vi "climb with joysticks.vi"   [LabVIEW 2012]
uses:
  <vilib>/Rock Robotics/WPI/Solenoid/WPI_SolenoidValue.ctl
  Robot Global Data.vi
  <vilib>/Rock Robotics/WPI/Solenoid/WPI_SolenoidSetEnum.vi
types:
  T1 = typedef "WPI_JoystickButtonState.ctl" = cluster{"Button 1":bool, "Button 2":bool, "Button 3":bool, "Button 4":bool, "Button 5":bool, "Button 6":bool, "Button 7":bool, "Button 8":bool, "Button 9":bool, "Button 10":bool, "Button 11":bool, "Button 12":bool}
  T2 = typedef "WPI_SolenoidValue.ctl" = enum16{"Off", "On", "Forward", "Reverse"}
  T3 = typedef "WPI_SolenoidDevRef.ctl" = cluster{"DevStatus":errorcluster, "Solenoid Module":T4, "Forward Solenoid Channel":T5, "Reverse Solenoid Channel":T5}
  T4 = typedef "FPGA_TypedefSolenoidModule.ctl" = enum16{"Solenoid Module 1", "Solenoid Module 2"}
  T5 = typedef "WPI_SolenoidChannel.ctl" = enum8{"Solenoid 1", "Solenoid 2", "Solenoid 3", "Solenoid 4", "Solenoid 5", "Solenoid 6", "Solenoid 7", "Solenoid 8", "Invalid"}
  T6 = typedef "WPI_MotorControlDeviceRef.ctl" = cluster{"DeviceStatus":errorcluster, "Type":enum16{"PWM", "CAN"}, "PWM":cluster{"Digital Module":T7, "PWM Channel":T8, "DeadBand":T9}, "CAN":cluster{"Device Number":u8, "Control Mode":T10, "Semaphore":T11, "Max Vout":dbl}, "Invert":bool, "TransformRef":T12, "InvTransformRef":T12}
  T7 = typedef "FPGA_TypedefDigitalModule.ctl" = enum16{"Digital Module 1", "Digital Module 2"}
  T8 = typedef "FPGA_DIOPWMChannel.ctl" = enum8{"PWM 1", "PWM 2", "PWM 3", "PWM 4", "PWM 5", "PWM 6", "PWM 7", "PWM 8", "PWM 9", "PWM 10", "Invalid"}
  T9 = typedef "WPI_PWMDeadband.ctl" = cluster{"Name":string, "maxPositivePwm":i32, "minPositivePwm":i32, "centerPwm":i32, "maxNegativePwm":i32, "minNegativePwm":i32, "angularRange":u16}
  T10 = typedef "WPI_CANJaguar_ControlMode.ctl" = enum8{"Percent VBus", "Current", "Speed", "Position", "Voltage"}
  T11 = typedef "Semaphore RefNum" = refnum<k1>
  T12 = typedef "WPI_PWMTransform_ConPane.ctl" = refnum<vi>
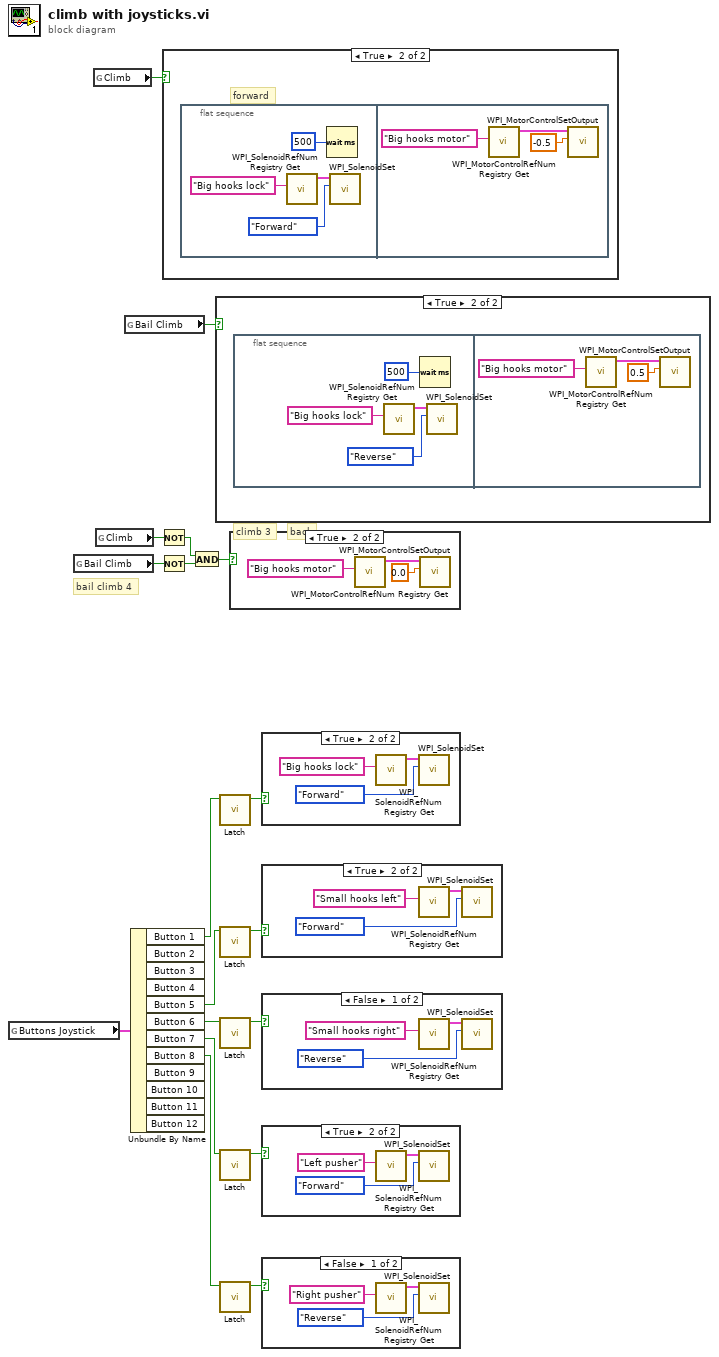
[diagram p0: block diagram]
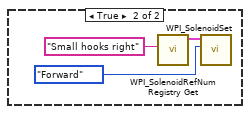
[diagram p2: hidden frame]
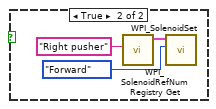
[diagram p3: hidden frame]
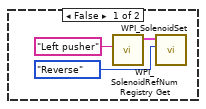
[diagram p4: hidden frame]
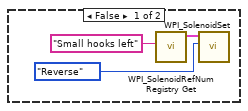
[diagram p5: hidden frame]
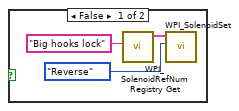
[diagram p6: hidden frame]
diagram:
  # "back"
  # "bail climb 4"
  # "climb 3"
  n1 = global read "Robot Global Data.vi" "Buttons Joystick"() -> (w11:T1)
  n2 = global read "Robot Global Data.vi" "Bail Climb"() -> (w13:bool)
  n3 = global read "Robot Global Data.vi" "Climb"() -> (w18:bool)
  n4 = global read "Robot Global Data.vi" "Climb"() -> (w15:bool)
  n5 = global read "Robot Global Data.vi" "Bail Climb"() -> (w17:bool)
  n6 = Unbundle By Name(w11) -> ("Button 1"=w10:bool, "Button 5"=w5:bool, "Button 6"=w1:bool, "Button 7"=w4:bool, "Button 8"=w3:bool)  [unwired: 7 out]
  n7 = Not(x=w15) -> (.not. x?=w14:bool)
  n8 = Not(x=w13) -> (.not. x?=w12:bool)
  n9 = case shown="True" w18 {
    frame False {
    }
    frame True {
      # "forward"
      n10 = flat-sequence {
        frame #0 {
          n11 = call <vilib>:"WPI_SolenoidRefNum Registry Get.vi"("refnum name"="Big hooks lock") -> ("SolenoidDevRef"=w21:T3)  [unwired: 9 in, 1 out]
          n12 = Wait (ms)(milliseconds to wait=u32 500) -> ()  [unwired: 1 out]
          n13 = call-poly <vilib>:"WPI_SolenoidSet.vi"("Value"=WPI_SolenoidValue."Forward", "SolenoidDevRef"=w21) -> ()  [unwired: 8 in, 2 out]
        }
        frame #1 {
          n14 = call <vilib>:"WPI_MotorControlRefNum Registry Get.vi"("refnum name"="Big hooks motor") -> ("MotorControlDevRef"=w25:T6)  [unwired: 9 in, 1 out]
          n15 = call <vilib>:"WPI_MotorControlSetOutput.vi"("Output"=-0.5, "MotorControlDevRef"=w25) -> ()  [unwired: 7 in, 3 out]
        }
      }
    }
  }
  n16 = And(x=w14, y=w12) -> (x .and. y?=w16:bool)
  n17 = case shown="True" w17 {
    frame False {
    }
    frame True {
      n18 = flat-sequence {
        frame #0 {
          n19 = call <vilib>:"WPI_SolenoidRefNum Registry Get.vi"("refnum name"="Big hooks lock") -> ("SolenoidDevRef"=w28:T3)  [unwired: 9 in, 1 out]
          n20 = Wait (ms)(milliseconds to wait=u32 500) -> ()  [unwired: 1 out]
          n21 = call-poly <vilib>:"WPI_SolenoidSet.vi"("Value"=WPI_SolenoidValue."Reverse", "SolenoidDevRef"=w28) -> ()  [unwired: 8 in, 2 out]
        }
        frame #1 {
          n22 = call <vilib>:"WPI_MotorControlRefNum Registry Get.vi"("refnum name"="Big hooks motor") -> ("MotorControlDevRef"=w32:T6)  [unwired: 9 in, 1 out]
          n23 = call <vilib>:"WPI_MotorControlSetOutput.vi"("Output"=0.5, "MotorControlDevRef"=w32) -> ()  [unwired: 7 in, 3 out]
        }
      }
    }
  }
  n24 = call "Latch.vi"("Input"=w10) -> ("Output"=w9:bool)  [unwired: 9 in]
  n25 = call "Latch.vi"("Input"=w5) -> ("Output"=w8:bool)  [unwired: 9 in]
  n26 = call "Latch.vi"("Input"=w1) -> ("Output"=w2:bool)  [unwired: 9 in]
  n27 = call "Latch.vi"("Input"=w4) -> ("Output"=w7:bool)  [unwired: 9 in]
  n28 = call "Latch.vi"("Input"=w3) -> ("Output"=w6:bool)  [unwired: 9 in]
  n29 = case shown="True" w16 {
    frame False {
    }
    frame True {
      n30 = call <vilib>:"WPI_MotorControlRefNum Registry Get.vi"("refnum name"="Big hooks motor") -> ("MotorControlDevRef"=w35:T6)  [unwired: 9 in, 1 out]
      n31 = call <vilib>:"WPI_MotorControlSetOutput.vi"("Output"=0.0, "MotorControlDevRef"=w35) -> ()  [unwired: 7 in, 3 out]
    }
  }
  n32 = case shown="True" w9 {
    frame False {
      n33 = call <vilib>:"WPI_SolenoidRefNum Registry Get.vi"("refnum name"="Big hooks lock") -> ("SolenoidDevRef"=w37:T3)  [unwired: 9 in, 1 out]
      n34 = call-poly <vilib>:"WPI_SolenoidSet.vi"("Value"=WPI_SolenoidValue."Reverse", "SolenoidDevRef"=w37) -> ()  [unwired: 8 in, 2 out]
    }
    frame True {
      n35 = call <vilib>:"WPI_SolenoidRefNum Registry Get.vi"("refnum name"="Big hooks lock") -> ("SolenoidDevRef"=w40:T3)  [unwired: 9 in, 1 out]
      n36 = call-poly <vilib>:"WPI_SolenoidSet.vi"("Value"=WPI_SolenoidValue."Forward", "SolenoidDevRef"=w40) -> ()  [unwired: 8 in, 2 out]
    }
  }
  n37 = case shown="True" w8 {
    frame False {
      n38 = call <vilib>:"WPI_SolenoidRefNum Registry Get.vi"("refnum name"="Small hooks left") -> ("SolenoidDevRef"=w43:T3)  [unwired: 9 in, 1 out]
      n39 = call-poly <vilib>:"WPI_SolenoidSet.vi"("Value"=WPI_SolenoidValue."Reverse", "SolenoidDevRef"=w43) -> ()  [unwired: 8 in, 2 out]
    }
    frame True {
      n40 = call <vilib>:"WPI_SolenoidRefNum Registry Get.vi"("refnum name"="Small hooks left") -> ("SolenoidDevRef"=w46:T3)  [unwired: 9 in, 1 out]
      n41 = call-poly <vilib>:"WPI_SolenoidSet.vi"("Value"=WPI_SolenoidValue."Forward", "SolenoidDevRef"=w46) -> ()  [unwired: 8 in, 2 out]
    }
  }
  n42 = case shown="False" w2 {
    frame False {
      n43 = call <vilib>:"WPI_SolenoidRefNum Registry Get.vi"("refnum name"="Small hooks right") -> ("SolenoidDevRef"=w49:T3)  [unwired: 9 in, 1 out]
      n44 = call-poly <vilib>:"WPI_SolenoidSet.vi"("Value"=WPI_SolenoidValue."Reverse", "SolenoidDevRef"=w49) -> ()  [unwired: 8 in, 2 out]
    }
    frame True {
      n45 = call <vilib>:"WPI_SolenoidRefNum Registry Get.vi"("refnum name"="Small hooks right") -> ("SolenoidDevRef"=w52:T3)  [unwired: 9 in, 1 out]
      n46 = call-poly <vilib>:"WPI_SolenoidSet.vi"("Value"=WPI_SolenoidValue."Forward", "SolenoidDevRef"=w52) -> ()  [unwired: 8 in, 2 out]
    }
  }
  n47 = case shown="True" w7 {
    frame False {
      n48 = call <vilib>:"WPI_SolenoidRefNum Registry Get.vi"("refnum name"="Left pusher") -> ("SolenoidDevRef"=w55:T3)  [unwired: 9 in, 1 out]
      n49 = call-poly <vilib>:"WPI_SolenoidSet.vi"("Value"=WPI_SolenoidValue."Reverse", "SolenoidDevRef"=w55) -> ()  [unwired: 8 in, 2 out]
    }
    frame True {
      n50 = call <vilib>:"WPI_SolenoidRefNum Registry Get.vi"("refnum name"="Left pusher") -> ("SolenoidDevRef"=w58:T3)  [unwired: 9 in, 1 out]
      n51 = call-poly <vilib>:"WPI_SolenoidSet.vi"("Value"=WPI_SolenoidValue."Forward", "SolenoidDevRef"=w58) -> ()  [unwired: 8 in, 2 out]
    }
  }
  n52 = case shown="False" w6 {
    frame False {
      n53 = call <vilib>:"WPI_SolenoidRefNum Registry Get.vi"("refnum name"="Right pusher") -> ("SolenoidDevRef"=w61:T3)  [unwired: 9 in, 1 out]
      n54 = call-poly <vilib>:"WPI_SolenoidSet.vi"("Value"=WPI_SolenoidValue."Reverse", "SolenoidDevRef"=w61) -> ()  [unwired: 8 in, 2 out]
    }
    frame True {
      n55 = call <vilib>:"WPI_SolenoidRefNum Registry Get.vi"("refnum name"="Right pusher") -> ("SolenoidDevRef"=w64:T3)  [unwired: 9 in, 1 out]
      n56 = call-poly <vilib>:"WPI_SolenoidSet.vi"("Value"=WPI_SolenoidValue."Forward", "SolenoidDevRef"=w64) -> ()  [unwired: 8 in, 2 out]
    }
  }
